vi "ReadUIParametersJSON.vi"(8 "error in":errorcluster, 11 "User interface JSON filepath":path=path "F:/Backup/ZenGage V1.3 Alpha/Configuration file/User Interface JSON.json") -> (0 "error out":errorcluster, 3 "UI JSON":T1)   [LabVIEW 2019, in "ZenGage v3.0 UI.lvclass"]
uses:
  ZenGage v3.0 UI.lvclass
  Type Definitions/JSON Read/UI JSON read cluster.ctl
panel:
  out "Error Message":string
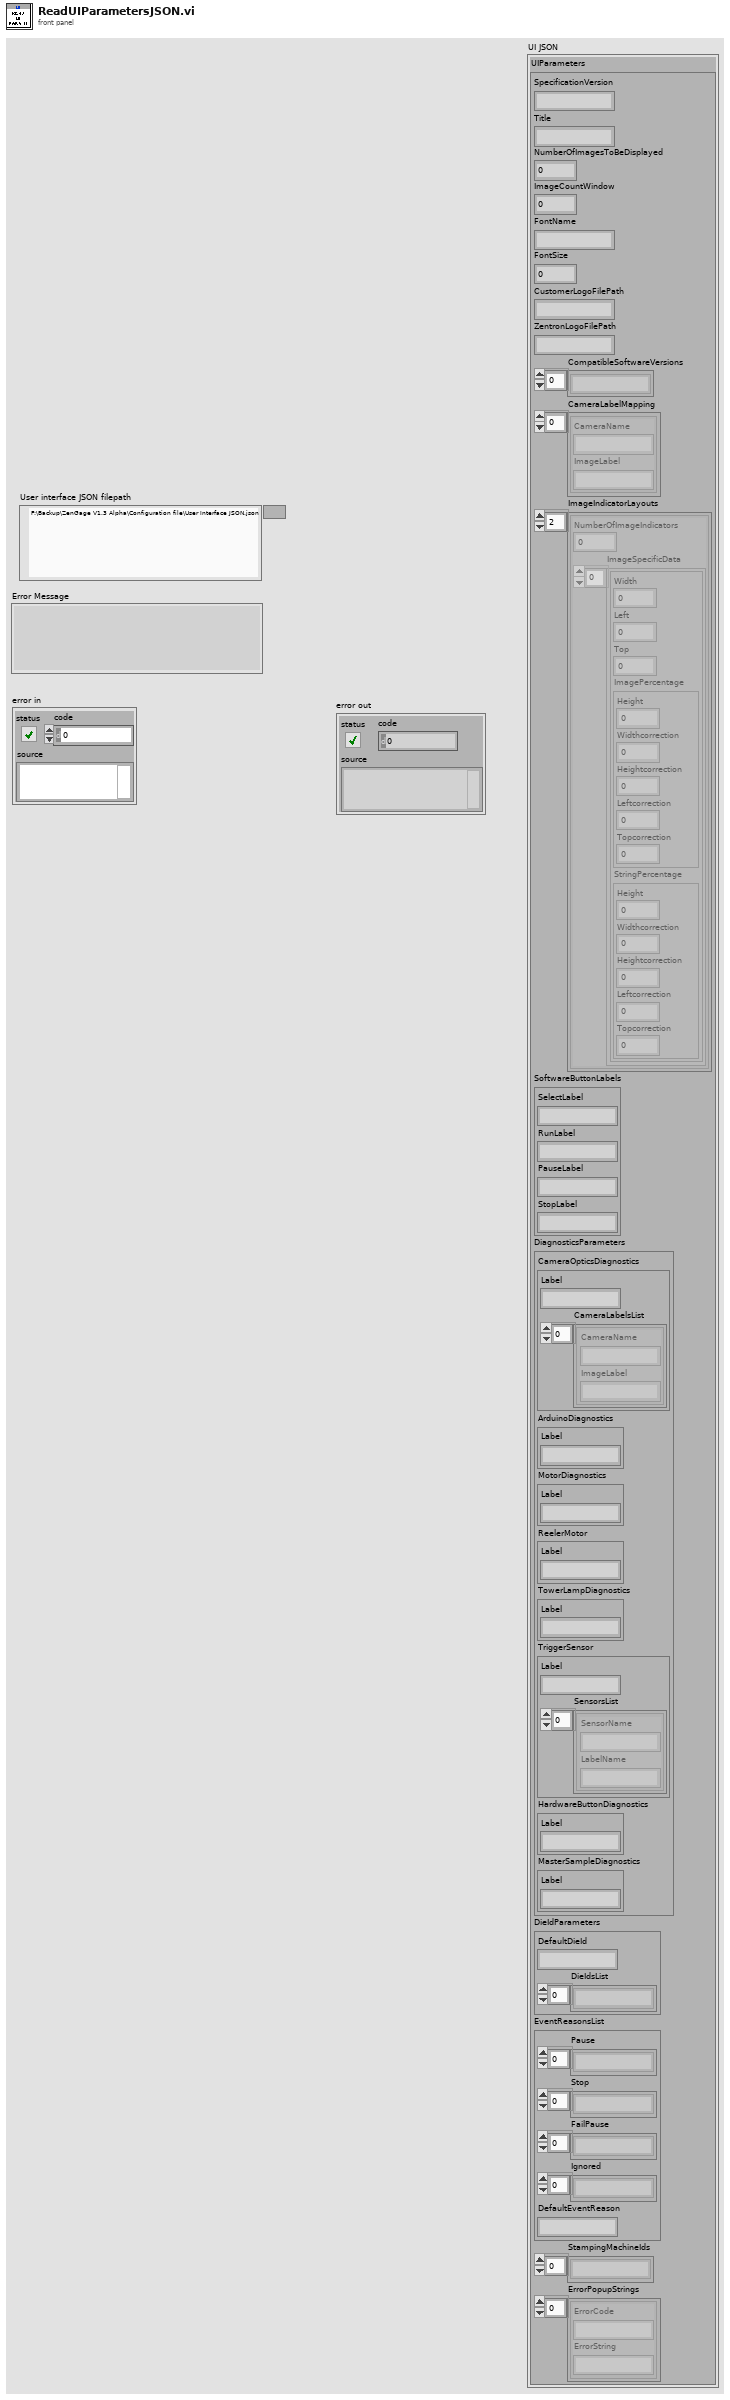
[diagram p1: front panel]
types:
  T1 = typedef "ZenGage v3.0 UI.lvclass/UI JSON read cluster.ctl" = cluster{"UIParameters":cluster{"SpecificationVersion":string, "Title":string, "NumberOfImagesToBeDisplayed":dbl, "ImageCountWindow":dbl, "FontName":string, "FontSize":dbl, "CustomerLogoFilePath":string, "ZentronLogoFilePath":string, "CompatibleSoftwareVersions":string[], "CameraLabelMapping":cluster{"CameraName":string, "ImageLabel":string}[], "ImageIndicatorLayouts":cluster{"NumberOfImageIndicators":dbl, "ImageSpecificData":cluster{"Width":dbl, "Left":dbl, "Top":dbl, "ImagePercentage":cluster{"Height":dbl, "Widthcorrection":i64, "Heightcorrection":i64, "Leftcorrection":dbl, "Topcorrection":dbl}, "StringPercentage":cluster{"Height":dbl, "Widthcorrection":i64, "Heightcorrection":dbl, "Leftcorrection":dbl, "Topcorrection":dbl}}[]}[], "SoftwareButtonLabels":cluster{"SelectLabel":string, "RunLabel":string, "PauseLabel":string, "StopLabel":string}, "DiagnosticsParameters":cluster{"CameraOpticsDiagnostics":cluster{"Label":string, "CameraLabelsList":cluster{"CameraName":string, "ImageLabel":string}[]}, "ArduinoDiagnostics":cluster{"Label":string}, "MotorDiagnostics":cluster{"Label":string}, "ReelerMotor":cluster{"Label":string}, "TowerLampDiagnostics":cluster{"Label":string}, "TriggerSensor":cluster{"Label":string, "SensorsList":cluster{"SensorName":string, "LabelName":string}[]}, "HardwareButtonDiagnostics":cluster{"Label":string}, "MasterSampleDiagnostics":cluster{"Label":string}}, "DieIdParameters":cluster{"DefaultDieId":string, "DieIdsList":string[]}, "EventReasonsList":cluster{"Pause":string[], "Stop":string[], "FailPause":string[], "Ignored":string[], "DefaultEventReason":string}, "StampingMachineIds":string[], "ErrorPopupStrings":cluster{"ErrorCode":string, "ErrorString":string}[]}}
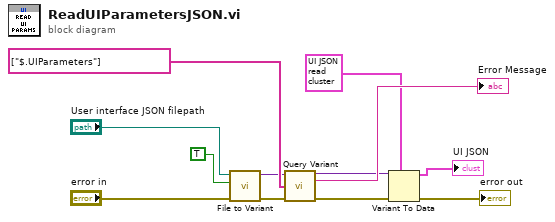
[diagram p0: block diagram]
diagram:
  n1 = call <vilib>:"File to Variant.vi"("JSON FilePath"="User interface JSON filepath", "Remove Comments?"=TRUE, "error in (no error)"="error in") -> ("JSON Variant"=w1:variant, "error out"=w7:errorcluster)  [unwired: 5 in, 1 out]
  n2 = call <vilib>:"Query Variant.vi"("VCluster in"=w1, "pathList"=string[] ["$.UIParameters"], "error IO"=w7) -> ("VCluster\n out"=w2:variant, "Error Message"=→"Error Message":string, "error out"=w10:errorcluster)  [unwired: 9 in, 1 out]
  n3 = Variant To Data(error in=w10, type=T1 {"UIParameters"={"SpecificationVersion"="", "Title"="", "NumberOfImagesToBeDisplayed"=0.0, "ImageCountWindow"=0.0, "FontName"="", "FontSize"=0.0, "CustomerLogoFilePath"="", "ZentronLogoFilePath"="", "CompatibleSoftwareVersions"=[], "CameraLabelMapping"=[], "ImageIndicatorLayouts"=[], "SoftwareButtonLabels"={"SelectLabel"="", "RunLabel"="", "PauseLabel"="", "StopLabel"=""}, "DiagnosticsParameters"={"CameraOpticsDiagnostics"={"Label"="", "CameraLabelsList"=[]}, "ArduinoDiagnostics"={"Label"=""}, "MotorDiagnostics"={"Label"=""}, "ReelerMotor"={"Label"=""}, "TowerLampDiagnostics"={"Label"=""}, "TriggerSensor"={"Label"="", "SensorsList"=[]}, "HardwareButtonDiagnostics"={"Label"=""}, "MasterSampleDiagnostics"={"Label"=""}}, "DieIdParameters"={"DefaultDieId"="", "DieIdsList"=[]}, "EventReasonsList"={"Pause"=[], "Stop"=[], "FailPause"=[], "Ignored"=[], "DefaultEventReason"=""}, "StampingMachineIds"=[], "ErrorPopupStrings"=[]}} ("UI JSON read cluster"), Variant=w2) -> (data=→"UI JSON":T1, error out=→"error out":errorcluster)
